vi "shutdown j1939.vi"(8 "error in":errorcluster, 10 "tag bus queues":T1, 11 "J1939 internal data":T2={"J1939 XNET Settings"={"XNET Database"="", "XNET Cluster"="", "CAN port"="", "Baud rate [Bd]"=0, "J1939 Network Address"=0, "Name"=0, "Termination"=0}, "j1939 queues"={"Processed Outgoing"=refnum, "Process Outgoing"=refnum, "stop notifier"=refnum, "error queue"=refnum, "active dtc"=refnum, "processed inc"=refnum}, "fgv references"={"BAM Buffer"=refnum, "CM Buffer"=refnum, "CM Gen"=refnum, "BAM Gen"=refnum, "Address Claims"=refnum, "RQST"=refnum, "scaling lut"=refnum, "data lut"=refnum, "cyclic scheduler"=refnum}, "frame in"="", "frame out"="", "timing"={"tb to j1939 queue timeout"=100, "j1939 to tb queue timeout"=100, "dtc loop period (ms)"=100, "CAN in loop period (ms)"=100, "process incoming queue timeout (ms)"=100, "Outgoing Write Decimation"=0, "process outgoing loop rate (ms)"=0, "periodic outgoing queue timeout (ms)"=10, "CAN out queue timeout (ms)"=100}}) -> (0 "error out":errorcluster, 3 "stop notifier":refnum<notifier>)   [LabVIEW 2013, in "J1939.lvlib"]
uses:
  J1939.lvlib
  Internals/API Types/Internal Data.ctl
  Internals/API Types/XNET Settings.ctl
  Internals/API Types/Setup Information Cluster.ctl
  Internals/API Types/CAN Outgoing Message Cluster.ctl
  Internals/API Types/Convert DTCs Cluster.ctl
  <vilib>/xnet/xnet.llb/XNET Frame CAN.ctl
  <vilib>/xnet/xnet.llb/XNET Frame Type CAN.ctl
  Internals/TP/TP List References.ctl
  Internals/BAM/BAM Buffer Connections List_Ref.ctl
  Internals/Connection Mode/Connection Mode Generation Connection Ref.ctl
  Internals/BAM/BAM Generation Connections List_Ref.ctl
  Internals/LUTs/J1939 Address Table Reference.ctl
  Internals/RQST/RQST Lookup Table Reference.ctl
  Internals/LUTs/J1939 Conversion Lookup Table Reference.ctl
  Internals/LUTs/J1939 Data Lookup Table Reference.ctl
  Internals/LUTs/Cyclic Frame Scheduler Lut Reference.ctl
  Configuration/TypeDefs/timing configuration.ctl
  Internals/API Types/Tag Bus Queues.ctl
  <vilib>/NI/Tag Bus/table/data table.ctl
  <vilib>/xnet/xnet.llb/XNET Database Close (Cluster).vi
  <vilib>/xnet/xnet.llb/XNET Database Close (Database).vi
  <vilib>/NI/Tag Bus/table/data table.lvlib
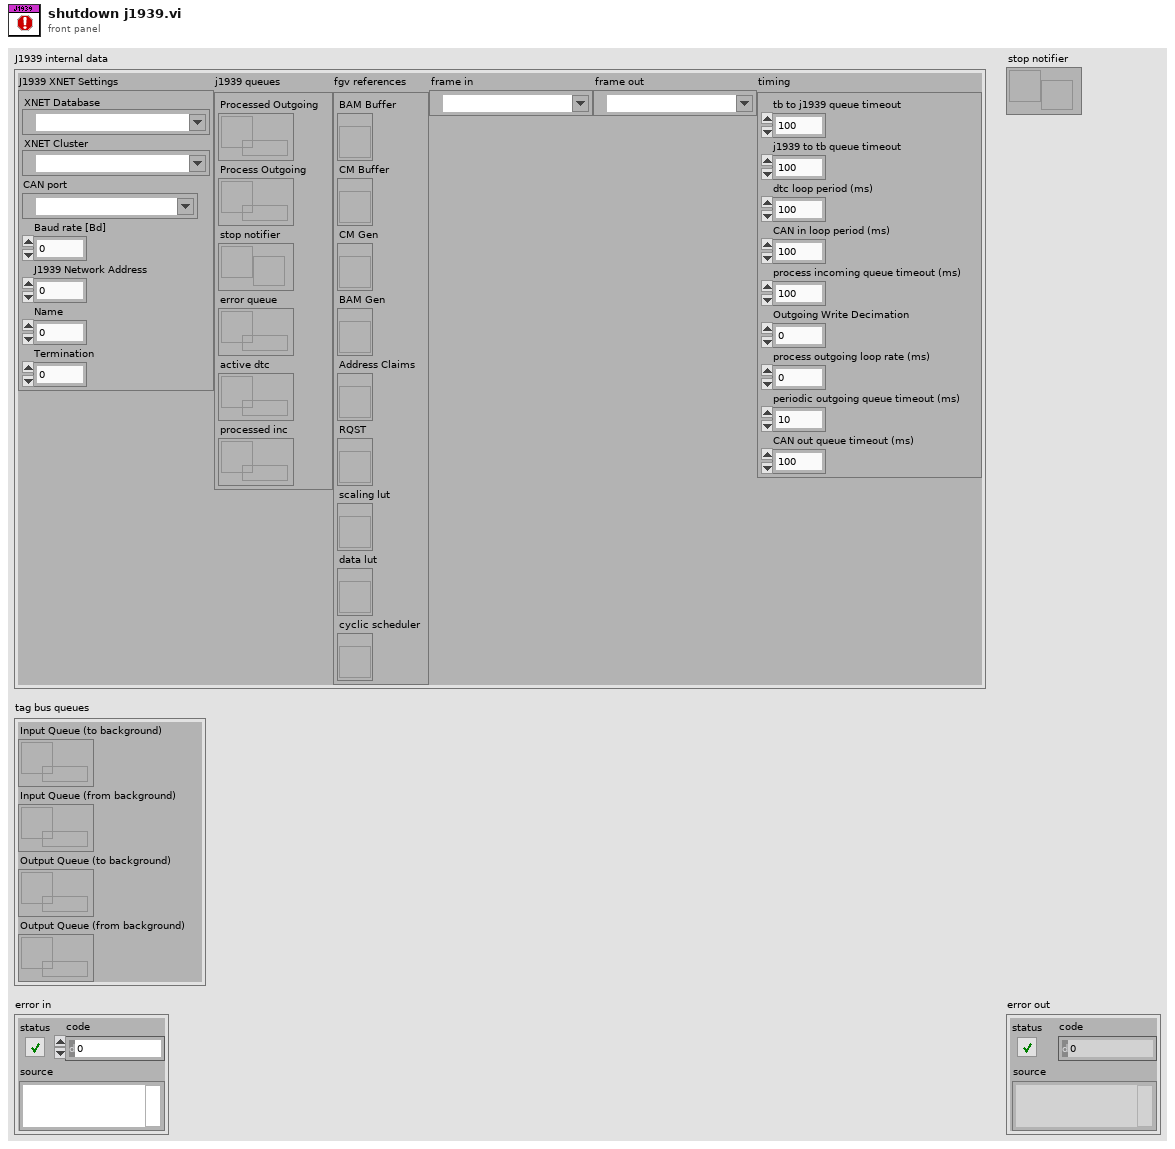
[diagram p1: front panel]
types:
  T1 = typedef "J1939.lvlib/Tag Bus Queues.ctl" = cluster{"Input Queue (to background)":refnum<queue>, "Input Queue (from background)":refnum<queue>, "Output Queue (to background)":refnum<queue>, "Output Queue (from background)":refnum<queue>}
  T2 = typedef "J1939.lvlib/Internal Data.ctl" = cluster{"J1939 XNET Settings":T3, "j1939 queues":T4, "fgv references":T5, "frame in":refnum<k21>, "frame out":refnum<k21>, "timing":T14}
  T3 = typedef "J1939.lvlib/XNET settings.ctl" = cluster{"XNET Database":refnum<k21>, "XNET Cluster":refnum<k21>, "CAN port":refnum<k21>, "Baud rate [Bd]":u32, "J1939 Network Address":u8, "Name":u64, "Termination":u32}
  T4 = typedef "J1939.lvlib/Setup Information Cluster.ctl" = cluster{"Processed Outgoing":refnum<queue>, "Process Outgoing":refnum<queue>, "stop notifier":refnum<notifier>, "error queue":refnum<queue>, "active dtc":refnum<queue>, "processed inc":refnum<queue>}
  T5 = typedef "J1939.lvlib/TP List References.ctl" = cluster{"BAM Buffer":T6, "CM Buffer":T6, "CM Gen":T7, "BAM Gen":T8, "Address Claims":T9, "RQST":T10, "scaling lut":T11, "data lut":T12, "cyclic scheduler":T13}
  T6 = typedef "J1939.lvlib/BAM Buffer Connections List_Ref.ctl" = refnum<vi>
  T7 = typedef "J1939.lvlib/Connection Mode Generation Connection Ref.ctl" = refnum<vi>
  T8 = typedef "J1939.lvlib/BAM Generation Connections List_Ref.ctl" = refnum<vi>
  T9 = typedef "J1939.lvlib/J1939 Address Table Reference.ctl" = refnum<vi>
  T10 = typedef "J1939.lvlib/RQST Lookup Table Reference.ctl" = refnum<vi>
  T11 = typedef "J1939.lvlib/J1939 Conversion Lookup Table Reference.ctl" = refnum<vi>
  T12 = typedef "J1939.lvlib/J1939 Data Lookup Table Reference.ctl" = refnum<vi>
  T13 = typedef "J1939.lvlib/cyclic frame scheduler lut reference.ctl" = refnum<vi>
  T14 = typedef "J1939.lvlib/timing configuration.ctl" = cluster{"tb to j1939 queue timeout":i32, "j1939 to tb queue timeout":i32, "dtc loop period (ms)":i32, "CAN in loop period (ms)":i32, "process incoming queue timeout (ms)":i32, "Outgoing Write Decimation":u32, "process outgoing loop rate (ms)":i32, "periodic outgoing queue timeout (ms)":i32, "CAN out queue timeout (ms)":i32}
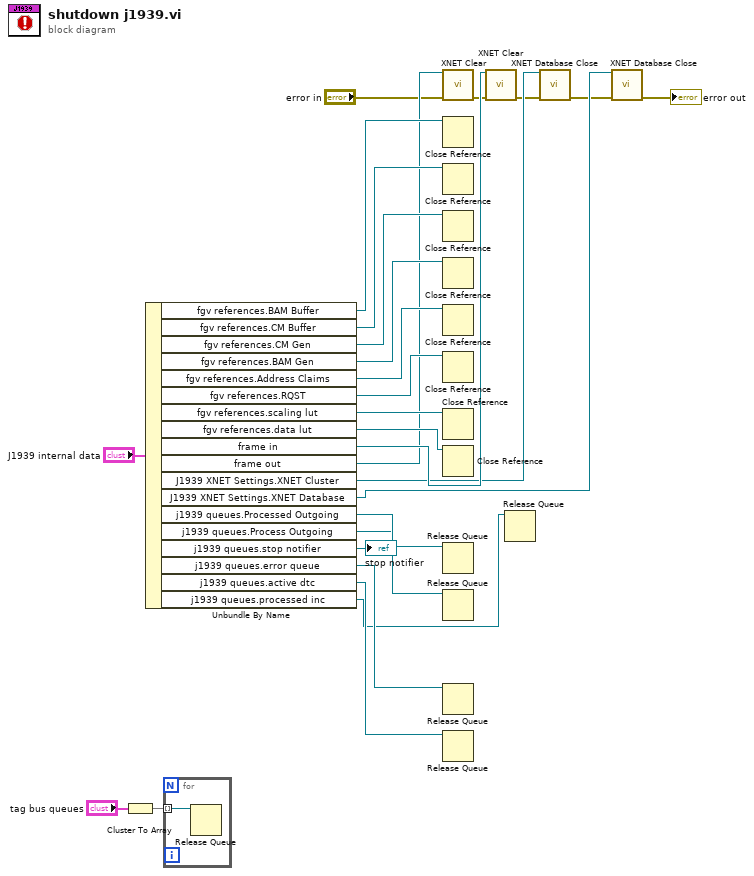
[diagram p0: block diagram]
diagram:
  n1 = Cluster To Array(cluster="tag bus queues") -> (array=w6:refnum<queue>[])
  n2 = Unbundle By Name("J1939 internal data") -> ("fgv references.BAM Buffer"=w25:T6, "fgv references.CM Buffer"=w24:T6, "fgv references.CM Gen"=w23:T7, "fgv references.BAM Gen"=w22:T8, "fgv references.Address Claims"=w21:T9, "fgv references.RQST"=w20:T10, "fgv references.scaling lut"=w19:T11, "fgv references.data lut"=w18:T12, "frame in"=w17:refnum<k21>, "frame out"=w16:refnum<k21>, "J1939 XNET Settings.XNET Cluster"=w15:refnum<k21>, "J1939 XNET Settings.XNET Database"=w14:refnum<k21>, "j1939 queues.Processed Outgoing"=w9:refnum<queue>, "j1939 queues.Process Outgoing"=w8:refnum<queue>, "j1939 queues.stop notifier"=→"stop notifier":refnum<notifier>, "j1939 queues.error queue"=w5:refnum<queue>, "j1939 queues.active dtc"=w4:refnum<queue>, "j1939 queues.processed inc"=w2:refnum<queue>)
  n3 = for {
    tunnel: w6 -> [w27] mode=indexing
    n4 = Release Queue(queue=w27) -> ()  [unwired: 2 in, 3 out]
  }
  n5 = call <vilib>:"XNET Clear.vi"("session in"=w16, "error in (no error)"="error in") -> ("error out"=w11:errorcluster)  [unwired: 13 in]
  n6 = Close Reference(reference=w25) -> ()  [unwired: 1 in, 1 out]
  n7 = Close Reference(reference=w24) -> ()  [unwired: 1 in, 1 out]
  n8 = Close Reference(reference=w23) -> ()  [unwired: 1 in, 1 out]
  n9 = Close Reference(reference=w22) -> ()  [unwired: 1 in, 1 out]
  n10 = Close Reference(reference=w21) -> ()  [unwired: 1 in, 1 out]
  n11 = Close Reference(reference=w20) -> ()  [unwired: 1 in, 1 out]
  n12 = Close Reference(reference=w19) -> ()  [unwired: 1 in, 1 out]
  n13 = Close Reference(reference=w18) -> ()  [unwired: 1 in, 1 out]
  n14 = Release Queue(queue=w9) -> ()  [unwired: 2 in, 3 out]
  n15 = Release Queue(queue=w8) -> ()  [unwired: 2 in, 3 out]
  n16 = Release Queue(queue=w5) -> ()  [unwired: 2 in, 3 out]
  n17 = Release Queue(queue=w4) -> ()  [unwired: 2 in, 3 out]
  n18 = call <vilib>:"XNET Clear.vi"("session in"=w17, "error in (no error)"=w11) -> ("error out"=w12:errorcluster)  [unwired: 13 in]
  n19 = Release Queue(queue=w2) -> ()  [unwired: 2 in, 3 out]
  n20 = call-poly <vilib>:"XNET Database Close.vi"("cluster in"=w15, "error in (no error)"=w12) -> ("error out"=w13:errorcluster)  [unwired: 13 in]
  n21 = call-poly <vilib>:"XNET Database Close.vi"("database in"=w14, "error in (no error)"=w13) -> ("error out"=→"error out":errorcluster)  [unwired: 13 in]
